vi "bubble_sort_final.vi"() -> ()   [LabVIEW 2016]
panel:
  out "Array 2":dbl[](array[numeric])
  in  "Array":dbl[](array[numeric])
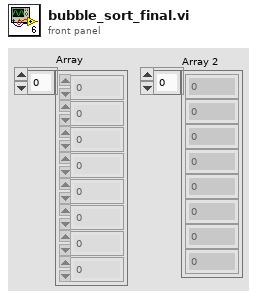
[diagram p1: front panel]
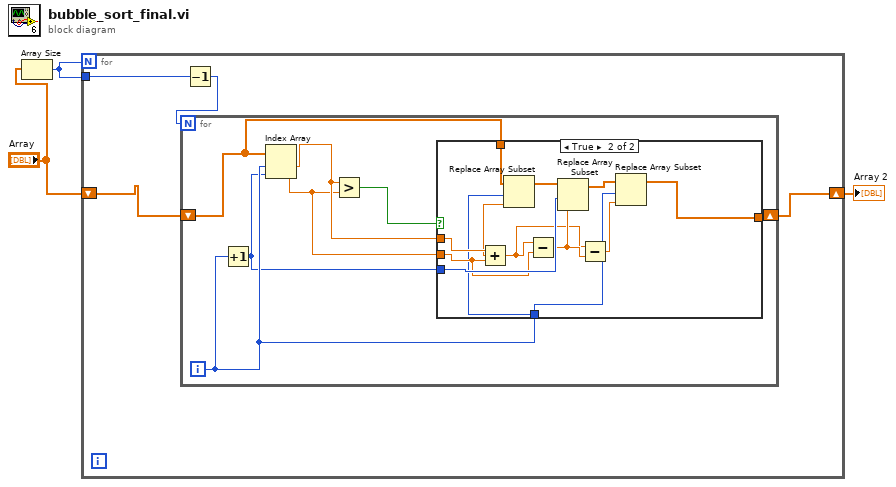
[diagram p0: block diagram]
diagram:
  n1 = Array Size(array="Array") -> (size(s)=w2:i32)
  n2 = for {
    N: w2 -> [_]
    shift-right: [w5] -> w1
    shift-left: "Array" -> [w6]
    tunnel: w2 -> [w4]
    n3 = Decrement(x=w4) -> (x-1=w7:i32)
    n4 = for {
      N: w7 -> [_]
      shift-right: [w9] -> w5
      shift-left: w6 -> [w8]
      i -> [w13]
      n5 = Increment(x=w13) -> (x+1=w10:i32)
      n6 = Index Array(array=w8, index #1=w13, index #2=w10) -> (element #1=w12:dbl, element #2=w11:dbl)
      n7 = Greater?(x=w12, y=w11) -> (0:w14:bool)
      n8 = case shown="True" w14 {
        tunnel: w13 -> [_ w20]
        tunnel: w12 -> [_ w25]
        tunnel: w11 -> [_ w22]
        tunnel: w10 -> [_ w23]
        tunnel: [w15 w16] -> w9
        tunnel: w8 -> [w15 w26]
        frame False {
        }
        frame True {
          n9 = Add(x=w25, y=w22) -> (x+y=w18:dbl)
          n10 = Replace Array Subset(array=w26, new element=w18, index=w20) -> (w24:dbl[])
          n11 = Subtract(x=w18, y=w22) -> (x-y=w19:dbl)
          n12 = Replace Array Subset(array=w24, new element=w19, index=w23) -> (w21:dbl[])
          n13 = Subtract(x=w18, y=w19) -> (x-y=w17:dbl)
          n14 = Replace Array Subset(array=w21, new element=w17, index=w20) -> (w16:dbl[])
        }
      }
    }
  }
  "Array 2" <- w1
